vi "Poll DMA.vi"(8 "error in":errorcluster, 10 "Injection.Results":T11 {"Shots"."Results"."Off-Stage Avg Current" format="%#.6g"; "Shots"."Results"."Total Voltage Pulses" format="%#.6g"; "Shots"."Results"."Off-Stage Min Current" format="%#.6g"; "Shots"."Results"."Off-Stage Max Current" format="%#.6g"}, 11 "Parameters":T1={"Name"="", "Rate.Hz"=0, "Injectors.Count"=0, "Injector.Timeout"=0.0, "Injector.Timer"=[], "Injector.Info"=[], "Events.Count"=[], "Event.Parameters"={"Shots"=0, "Shot.InitialVoltage"=0.0, "Shot.Stages"=0, "Stages"=[{"Stage.Dwell.Level"=0.0, "PullIn.Type"=enum."Pull In Transition Dwells", "PullIn.Level"=0.0, "Transition.Type"=enum."Stage Transition Voltage Level", "Transition.Level"=0.0}]}, "DMA.Ref"=refnum, "Waveform.Refs"=[], "Waveform.Sessions"=[], "Waveform.Enable"=refnum, "FPGA.Status"=refnum, "Search.Data"=refnum, "Results.Data"=refnum, "Results.Values"=[], "Results.Selections"=[]}) -> (0 "error out":errorcluster, 1 "Elements Remaining":u32, 3 "Parameters":T1={"Name"="", "Rate.Hz"=0, "Injectors.Count"=0, "Injector.Timeout"=0.0, "Injector.Timer"=[], "Injector.Info"=[], "Events.Count"=[], "Event.Parameters"={"Shots"=0, "Shot.InitialVoltage"=0.0, "Shot.Stages"=0, "Stages"=[{"Stage.Dwell.Level"=0.0, "PullIn.Type"=enum."Pull In Transition Dwells", "PullIn.Level"=0.0, "Transition.Type"=enum."Stage Transition Voltage Level", "Transition.Level"=0.0}]}, "DMA.Ref"=refnum, "Waveform.Refs"=[], "Waveform.Sessions"=[], "Waveform.Enable"=refnum, "FPGA.Status"=refnum, "Search.Data"=refnum, "Results.Data"=refnum, "Results.Values"=[], "Results.Selections"=[]})   [LabVIEW 2015, in "Fuel Injection Addon Engine.lvlib"]
uses:
  Fuel Injection Addon Engine.lvlib
  Types/Injector Event Data Cluster.ctl
  RT Analysis/Controls/Shot Information Control.ctl
  Types/Stage.Measurements.ctl
  Types/Async Parameters.ctl
  Shared/Types/Injector info.ctl
  Shared/Types/Shot.Parameters.ctl
  Shared/Types/Stage.Parameters.ctl
  Shared/Types/Stage.PullIn.Types.ctl
  Shared/Types/Stage.Transition.Types.ctl
  <vilib>/NI Veristand/Custom Device API/Waveform Data Reference.ctl
  <vilib>/NI VeriStand/Custom Device Waveform API/Single Waveform Write (DBL)/Single Waveform Write (DBL).lvclass
  <vilib>/NI/NIVS Inline Async API/_Data Access Engine/Data Access Engine/Types/Read.DVR.ctl
  <vilib>/NI/NIVS Inline Async API/_Data Access Engine/Access Type Classes/Read/Read.lvclass
  <vilib>/NI/NIVS Inline Async API/_Data Access Engine/Data Access Engine/Types/Write.DVR.ctl
  <vilib>/NI/NIVS Inline Async API/_Data Access Engine/Access Type Classes/Write/Write.lvclass
  Shared/Types/Analysis.Channels.Select.ctl
  <vilib>/NI/NIVS Inline Async API/_Data Access Engine/Access Type Classes/Read/Read.lvclass/Read.ctl
  <vilib>/NI VeriStand/Custom Device Waveform API/Waveform Session.lvclass/Waveform Session.ctl
  <vilib>/NI VeriStand/Custom Device Waveform API/Single Waveform Write (DBL)/Single Waveform Write (DBL).lvclass/Single Waveform Write (DBL).ctl
  <vilib>/NI VeriStand/Custom Device Waveform API/Internal Comm Classes/WPL Comm/WPL Comm (1D DBL)/WPL Comm (1D DBL).lvclass/WPL Comm (1D DBL).ctl
  <vilib>/NI VeriStand/Custom Device Waveform API/Internal Comm Classes/WPL Comm/WPL Comm.lvclass/WPL Comm.ctl
  <vilib>/NI/NIVS Inline Async API/_Data Access Engine/Access Type Classes/Write/Write.lvclass/Write.ctl
  Waveform Write.vi
  Stages.GetValues.vi
  Pack Data and Write to Inline.vi
  RT Analysis/subVIs/Build Event from Shots.vi
  Parse Injection Data.vi
  <vilib>/NI Veristand/Custom Device Waveform API/NI VeriStand - Write Waveform(s).vi
  <vilib>/NI Veristand/Custom Device Waveform API/Single Waveform Write (DBL)/NI VeriStand - Write Single Waveform (DBL).vi
  <vilib>/NI/NIVS Inline Async API/_Data Access Engine/Data Access Engine/Methods/Data.Processes.Execute.vi
  <vilib>/NI/NIVS Inline Async API/_Data Access Engine/Data Access Engine/Methods/Read.Data.vi
  Build Result Array from Shots.vi
  <vilib>/NI/NIVS Inline Async API/_Data Access Engine/Data Access Engine/Methods/Write.Data.vi
  RT Analysis/subVIs/Calculate Voltage Magnitude Measurements.vi
  RT Analysis/subVIs/Calculate Current Magnitude Measurements.vi
  <vilib>/NI Veristand/Custom Device Waveform API/Internal Comm Classes/WPL Comm/WPL Comm (1D DBL)/Comm_write 1d dbl.vi
  <vilib>/NI Veristand/Custom Device Waveform API/Read Sample offset DVR.vi
  <vilib>/NI Veristand/Custom Device Waveform API/Check Opened.vi
  <vilib>/NI/NIVS Inline Async API/_Data Access Engine/Access Type Classes/Read/Read.ProcessData.vi
  <vilib>/NI/NIVS Inline Async API/_Data Access Engine/Access Type Classes/Write/Write.ProcessData.vi
  RT Analysis/subVIs/Calculate Hold-In Voltage Measurements.vi
  RT Analysis/subVIs/Calculate Hold-In Measurements.vi
  <vilib>/Analysis/baseanly.llb/Mean.vi
  <vilib>/Analysis/baseanly.llb/Mean (DBL).vi
  <vilib>/NI Veristand/Custom Device Waveform API/Internal Comm Classes/WPL Comm/Direct Send WPL Command.vi
  <vilib>/NI Veristand/Custom Device Waveform API/Internal Comm Classes/WPL Comm/Convert Q Error to Shutdown Error.vi
  Shared/Constants.vi
  <vilib>/Analysis/8numeric.llb/Peak Detector.vi
  RT.Stages.Find.vi
  <vilib>/Utility/error.llb/Error Cluster From Error Code.vi
  <vilib>/rvi/errors/niLvFpgaAdjustHostInterfaceError.vi
  <vilib>/rvi/interface/nirviMethod/nirviMethod.xnode
  <vilib>/FPGAPlugInAG/Dynamic/niLvFpga_ReadFifo_Dynamic.vi
  <vilib>/rvi/errors/niLvFpgaMergeErrorWithErrorCode.vi
  Shared/Fuel Injection Addon Shared.lvlib
  <vilib>/NI VeriStand/Custom Device API/Custom Device API.lvlib
  <vilib>/NI/NIVS Inline Async API/_Data Access Engine/Data Access Engine/Data Access Engine.lvclass
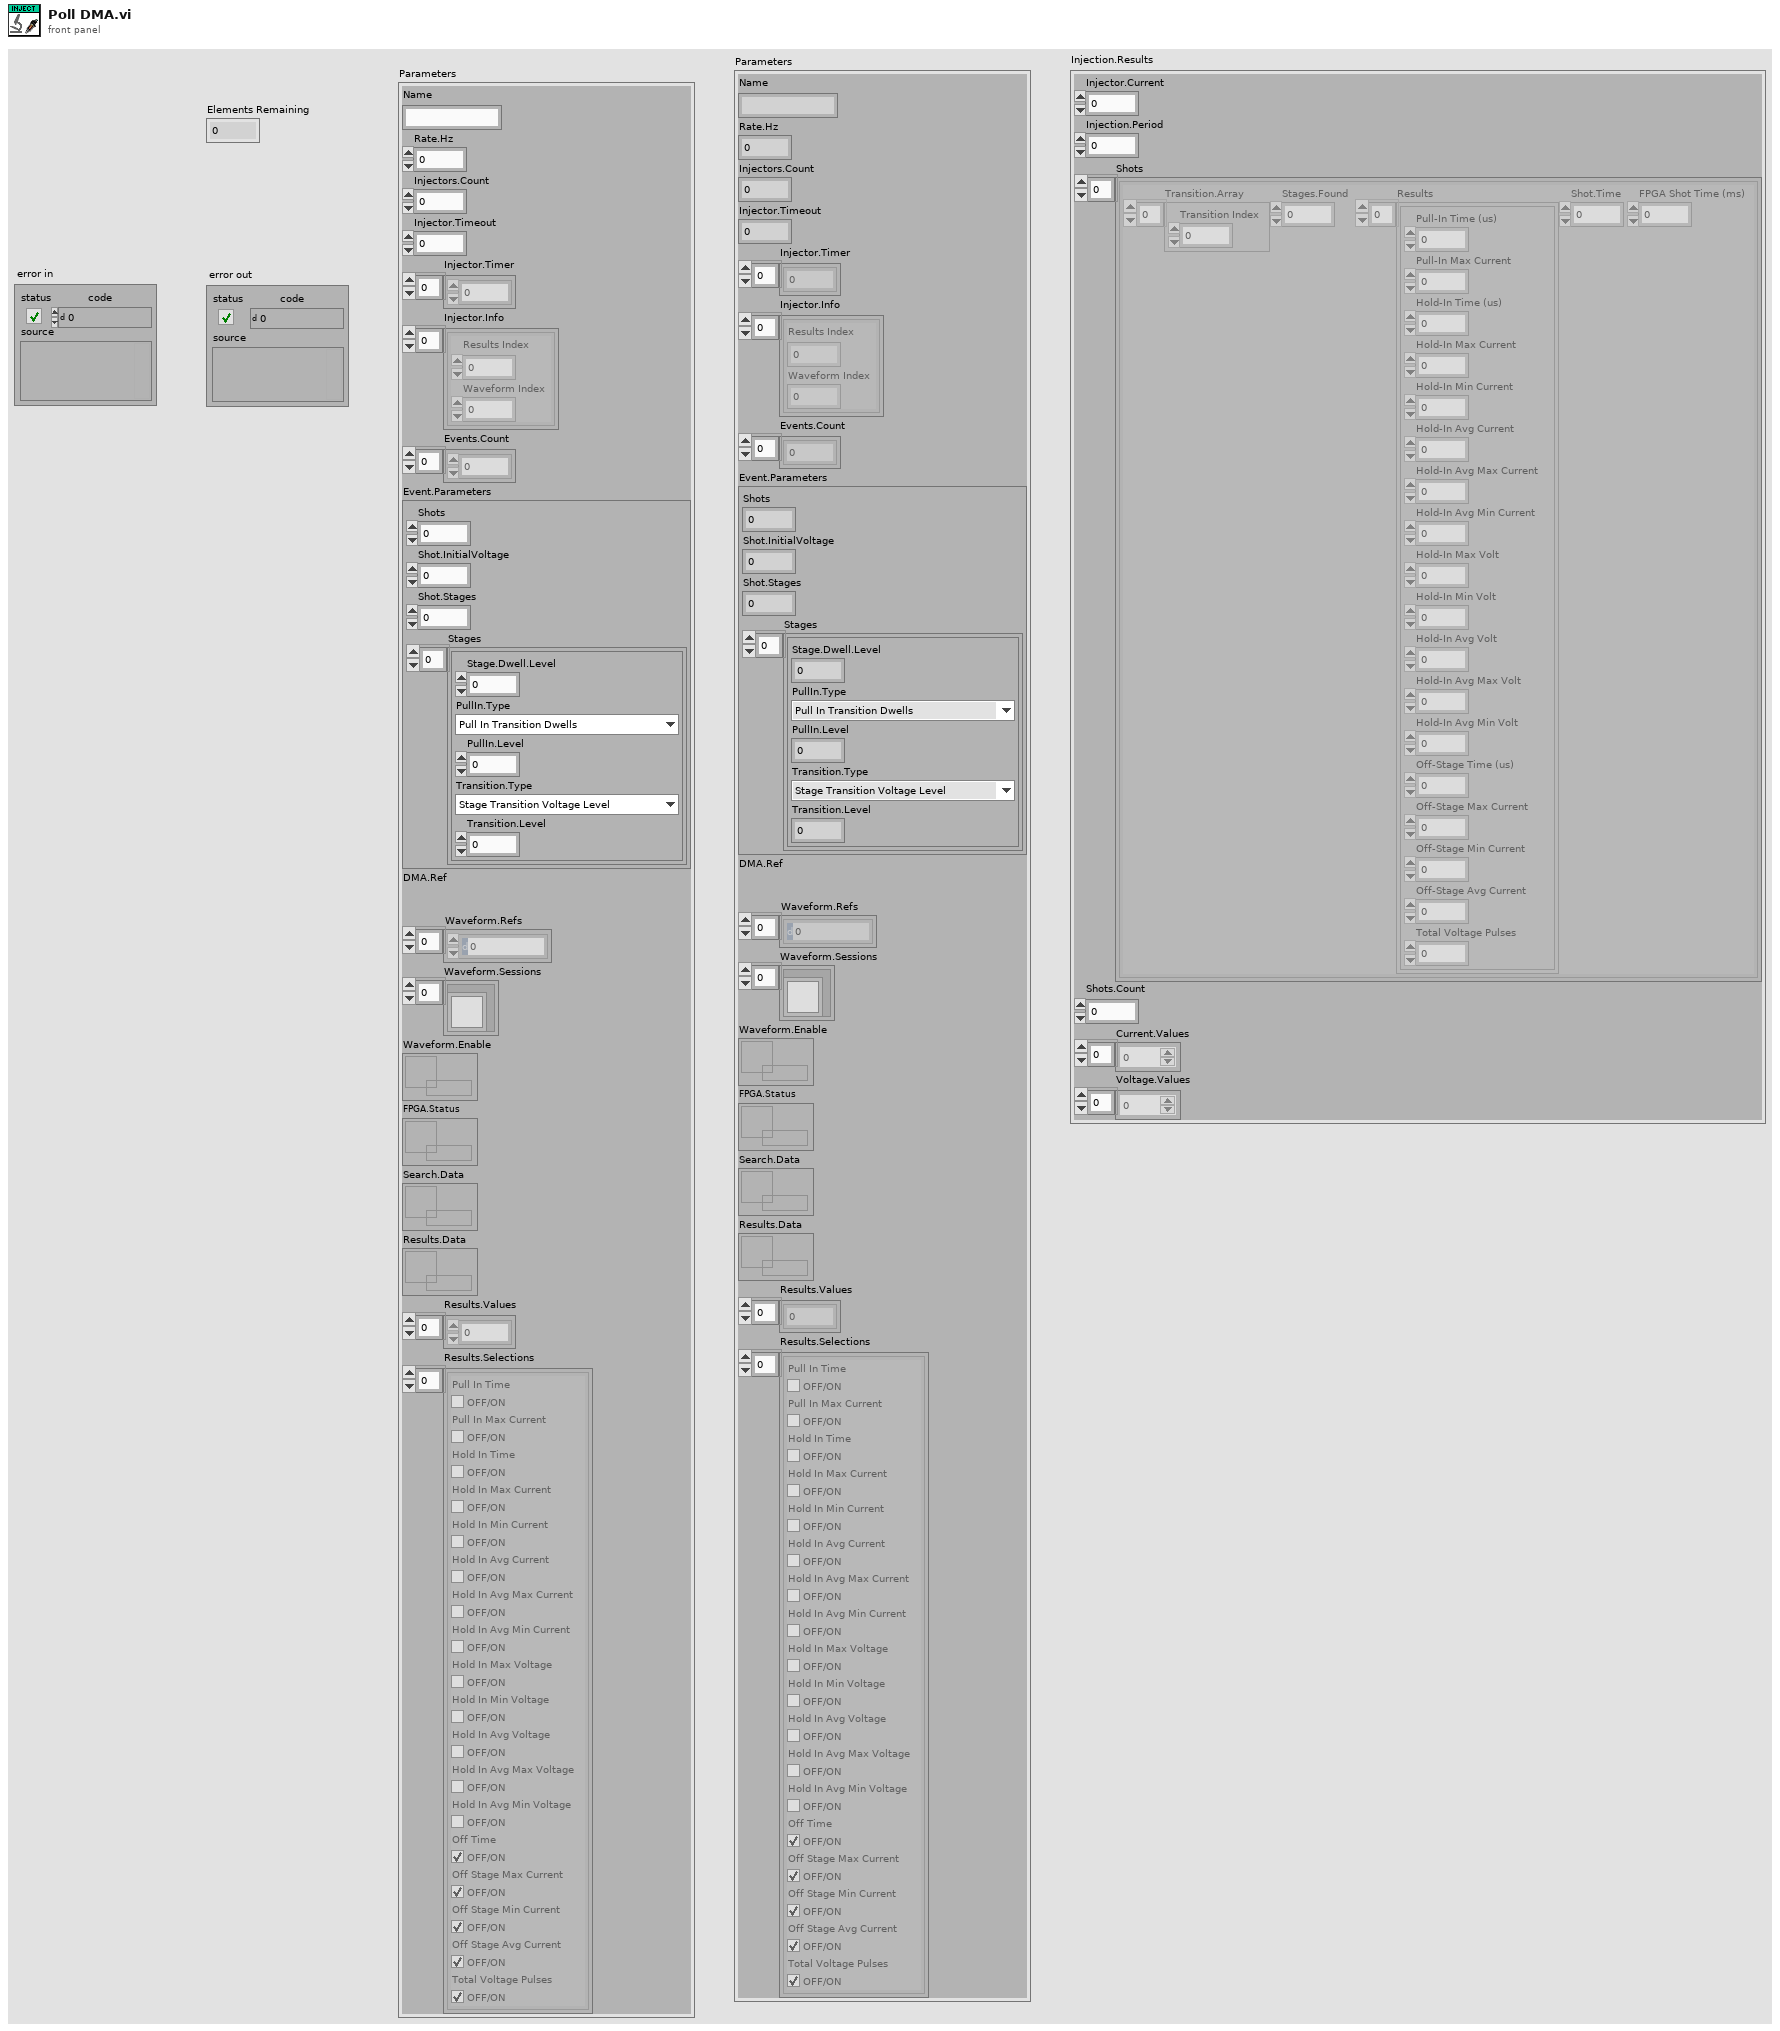
[diagram p1: front panel]
types:
  T1 = typedef "Fuel Injection Addon Engine.lvlib/Async Parameters.ctl" = cluster{"Name":string, "Rate.Hz":u32, "Injectors.Count":u8, "Injector.Timeout":dbl, "Injector.Timer":u32[], "Injector.Info":T2[], "Events.Count":u64[], "Event.Parameters":T3, "DMA.Ref":refnum<k20>, "Waveform.Refs":T7[], "Waveform.Sessions":refnum<class "Single Waveform Write (DBL).lvclass">[], "Waveform.Enable":T8, "FPGA.Status":T9, "Search.Data":T8, "Results.Data":T9, "Results.Values":dbl[], "Results.Selections":T10[]}
  T2 = typedef "Fuel Injection Addon Shared.lvlib/Injector info.ctl" = cluster{"Results Index":i32, "Waveform Index":i32}
  T3 = typedef "Fuel Injection Addon Shared.lvlib/Shot.Parameters.ctl" = cluster{"Shots":u32, "Shot.InitialVoltage":dbl, "Shot.Stages":u32, "Stages":T4[]}
  T4 = typedef "Fuel Injection Addon Shared.lvlib/Stage.Parameters.ctl" = cluster{"Stage.Dwell.Level":dbl, "PullIn.Type":T5, "PullIn.Level":dbl, "Transition.Type":T6, "Transition.Level":dbl}
  T5 = typedef "Fuel Injection Addon Shared.lvlib/Stage.PullIn.Types.ctl" = enum8{"Pull In Transition Dwells", "Pull In Transition Current Drop"}
  T6 = typedef "Fuel Injection Addon Shared.lvlib/Stage.Transition.Types.ctl" = enum8{"Stage Transition Dwell Time", "Stage Transition Voltage Level", "Stage Transition Current Drop"}
  T7 = typedef "Custom Device API.lvlib/Waveform Data Reference.ctl" = i32
  T8 = typedef "Data Access Engine.lvlib/Data Access Engine.lvclass/Read.DVR.ctl" = refnum<data-value>
  T9 = typedef "Data Access Engine.lvlib/Data Access Engine.lvclass/Write.DVR.ctl" = refnum<data-value>
  T10 = typedef "Fuel Injection Addon Shared.lvlib/Analysis.Channels.Select.ctl" = cluster{"Pull In Time":bool, "Pull In Max Current":bool, "Hold In Time":bool, "Hold In Max Current":bool, "Hold In Min Current":bool, "Hold In Avg Current":bool, "Hold In Avg Max Current":bool, "Hold In Avg Min Current":bool, "Hold In Max Voltage":bool, "Hold In Min Voltage":bool, "Hold In Avg Voltage":bool, "Hold In Avg Max Voltage":bool, "Hold In Avg Min Voltage":bool, "Off Time":bool, "Off Stage Max Current":bool, "Off Stage Min Current":bool, "Off Stage Avg Current":bool, "Total Voltage Pulses":bool}
  T11 = typedef "Fuel Injection Addon Engine.lvlib/Injector Event Data Cluster.ctl" = cluster{"Injector.Current":i16, "Injection.Period":dbl, "Shots":T12[], "Shots.Count":i32, "Current.Values":dbl[], "Voltage.Values":dbl[]}
  T12 = typedef "Fuel Injection Addon Engine.lvlib/Shot Information Control.ctl" = cluster{"Transition.Array":i32[], "Stages.Found":u16, "Results":T13[], "Shot.Time":dbl, "FPGA Shot Time (ms)":dbl}
  T13 = typedef "Fuel Injection Addon Engine.lvlib/Stage.Measurements.ctl" = cluster{"Pull-In Time (us)":dbl, "Pull-In Max Current":dbl, "Hold-In Time (us)":dbl, "Hold-In Max Current":dbl, "Hold-In Min Current":dbl, "Hold-In Avg Current":dbl, "Hold-In Avg Max Current":dbl, "Hold-In Avg Min Current":dbl, "Hold-In Max Volt":dbl, "Hold-In Min Volt":dbl, "Hold-In Avg Volt":dbl, "Hold-In Avg Max Volt":dbl, "Hold-In Avg Min Volt":dbl, "Off-Stage Time (us)":dbl, "Off-Stage Max Current":dbl, "Off-Stage Min Current":dbl, "Off-Stage Avg Current":dbl, "Total Voltage Pulses":dbl}
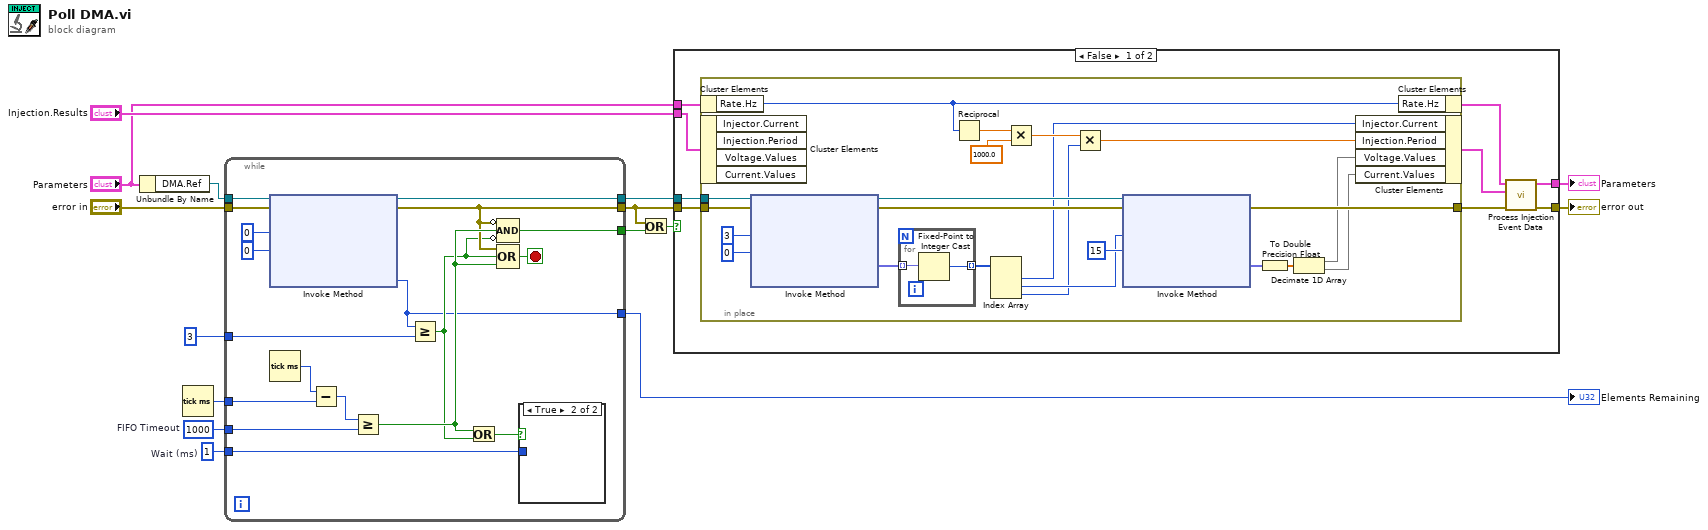
[diagram p0: block diagram]
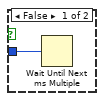
[diagram p3: hidden frame]
diagram:
  w3 = u32 1  # Wait (ms)
  w4 = u32 1000  # FIFO Timeout
  n1 = Unbundle By Name("Parameters") -> ("DMA.Ref"=w7:refnum<k20>)
  n2 = Tick Count (ms)() -> (millisecond timer value=w14:u32)
  n3 = while {
    tunnel: "error in" -> [w33]
    tunnel: w3 -> [w32]
    tunnel: w14 -> [w29]
    tunnel: w4 -> [w27]
    tunnel: [w25] -> w10
    tunnel: [w20] -> w11
    tunnel: [w19] -> w12
    tunnel: w7 -> [w23]
    tunnel: u32 3 ("Number of Elements") -> [w17]
    tunnel: [w16] -> w1
    stop <- w24 stop-if-true
    n4 = xnode "Invoke Method"("FPGA VI Reference In"=w23, "error in"=w33, "Number of Elements"=u32 0, "Timeout (ms)"=0) -> ("FPGA VI Reference Out"=w25:refnum<k20>, "error out"=w20:errorcluster, "Elements Remaining"=w16:u32)  [unwired: 1 out]
    n5 = Tick Count (ms)() -> (millisecond timer value=w30:u32)
    n6 = Subtract(x=w30, y=w29) -> (x-y=w28:u32)
    n7 = Greater Or Equal?(x=w28, y=w27) -> (x >= y?=w21:bool)
    n8 = Greater Or Equal?(x=w16, y=w17) -> (x >= y?=w18:bool)
    n9 = Or(x=w21, y=w18) -> (x .or. y?=w26:bool)
    n10 = Compound Arithmetic op=AND(invert w20, w21, invert w18) -> (w19:bool)
    n11 = Compound Arithmetic op=OR(w20, w18, w21) -> (w24:bool)
    n12 = case shown="True" w26 {
      tunnel: w32 -> [w34 _]
      frame False {
        n13 = Wait Until Next ms Multiple(millisecond multiple=w34) -> ()  [unwired: 1 out]
      }
      frame True {
      }
    }
  }
  "Elements Remaining" <- w1
  n14 = Or(x=w11, y=w12) -> (x .or. y?=w13:bool)
  n15 = case shown="False" w13 {
    tunnel: w11 -> [w42 w69]
    tunnel: w10 -> [w43 _]
    tunnel: [w40 w69] -> w8
    tunnel: "Injection.Results" -> [w36 _]
    tunnel: "Parameters" -> [w38 w68]
    tunnel: [w39 w68] -> w5
    frame False {
      n16 = in-place {
        in-place-border: w43 -> [w65]
        in-place-border: w42 -> [w64]
        in-place-border: [w57] -> w41
        n17 = in-place-cluster #1(w38) -> ("Rate.Hz"=w49:u32)
        n18 = in-place-cluster #2(w36) -> ()  [unwired: 4 out]
        n19 = xnode "Invoke Method"("FPGA VI Reference In"=w65, "error in"=w64, "Number of Elements"=u32 3, "Timeout (ms)"=0) -> ("FPGA VI Reference Out"=w60:refnum<k20>, "error out"=w59:errorcluster, "Data"=w62:fxp<+/-,32,8>[])  [unwired: 1 out]
        n20 = for {
          tunnel: w62 -> [w67] mode=indexing
          tunnel: [w66] -> w61 mode=indexing
          n21 = Fixed-Point to Integer Cast(1:w67) -> (0:w66:i32)
        }
        n22 = Reciprocal(x=w49) -> (1/x=w54:dbl)
        n23 = Index Array(array=w61) -> (element #1=w48:i32, element #2=w52:i32, element #3=w51:i32)  [unwired: 3 in]
        n24 = Multiply(x=w54, y=1000.0) -> (x*y=w53:dbl)
        n25 = Multiply(x=w53, y=w51) -> (x*y=w47:dbl)
        n26 = xnode "Invoke Method"("FPGA VI Reference In"=w60, "error in"=w59, "Number of Elements"=w52, "Timeout (ms)"=15) -> ("error out"=w57:errorcluster, "Data"=w56:fxp<+/-,32,8>[])  [unwired: 2 out]
        n27 = To Double Precision Float(number=w56) -> (double precision float=w50:dbl[])
        n28 = Decimate 1D Array(w50) -> (w46:dbl[], w45:dbl[])
        n29 = in-place-cluster #2("Injector.Current"=w48, "Injection.Period"=w47, "Voltage.Values"=w46, "Current.Values"=w45) -> (w35:T11)
        n30 = in-place-cluster #1("Rate.Hz"=w49) -> (w37:T1)
      }
      n31 = call "Process Injection Event Data.vi"("error in (no error)"=w41, "Injection.Results"=w35, "Parameters"=w37) -> ("error out"=w40:errorcluster, "Parameters"=w39:T1)  [unwired: 7 in]
    }
    frame True {
    }
  }
  "error out" <- w8
  "Parameters" <- w5
